vi "Check moving.vi"(8 "error in (no error)":errorcluster, 11 "ICS in":refnum<class "ICS.lvclass">) -> (0 "error out":errorcluster, 2 "in motion":bool, 3 "ICS out":refnum<class "ICS.lvclass">)   [LabVIEW 2018, in "ICS.lvclass"]
uses:
  ICS.lvclass
  ICS.lvclass/ICS.ctl
  Motor/Motor.lvclass
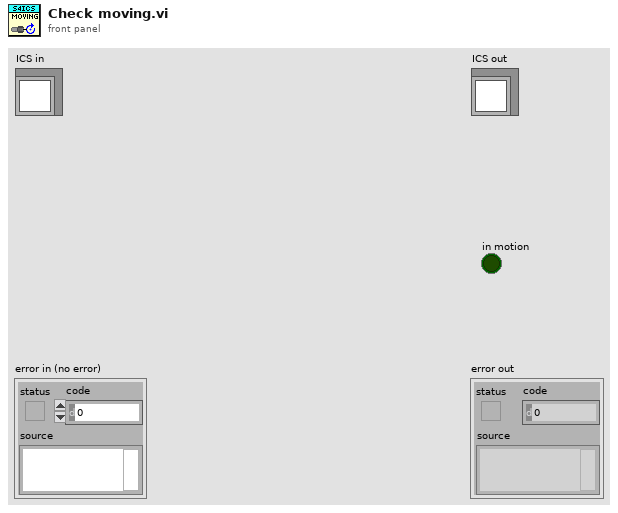
[diagram p1: front panel]
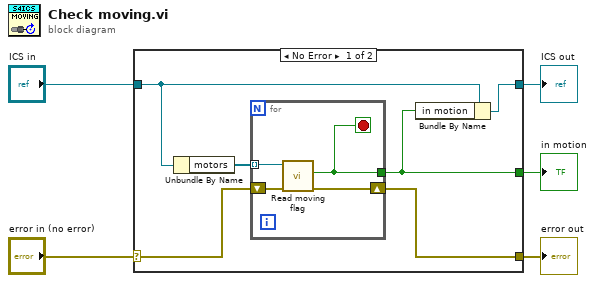
[diagram p0: block diagram]
diagram:
  n1 = case shown="No Error" "error in (no error)" {
    selector: "error in (no error)" -> [w10 w16]
    tunnel: [w9 w16] -> w4
    tunnel: [w6 w17] -> w2
    tunnel: "ICS in" -> [w8 w17]
    tunnel: [w7 _] -> w1
    frame No Error {
      n2 = Unbundle By Name(w8) -> ("motors"=w11:refnum<class "Motor.lvclass">[])
      n3 = for {
        tunnel: w11 -> [w15] mode=indexing
        shift-right: [w12] -> w9
        shift-left: w10 -> [w14]
        tunnel: [w13] -> w7
        stop <- w13 stop-if-true
        n4 = call-dynamic "Read moving flag.vi"("error in (no error)"=w14, "Motor in"=w15) -> ("error out"=w12:errorcluster, "moving"=w13:bool)  [unwired: 7 in, 1 out]
      }
      n5 = Bundle By Name(cluster=w8, "in motion"=w7) -> (w6:refnum<class "ICS.lvclass">)
    }
    frame Error {
    }
  }
  "error out" <- w4
  "ICS out" <- w2
  "in motion" <- w1
